vi "CAN Write.vi"(8 "error in (no error)":errorcluster, 10 "MessageBuffer":T1={"ID"=261, "MSGTYPE"=0, "LEN"=8, "DATA[0]"=37, "DATA[1]"=80, "DATA[2]"=37, "DATA[3]"=80, "DATA[4]"=37, "DATA[5]"=80, "DATA[6]"=37, "DATA[7]"=80} {"ID" format="%x"; "MSGTYPE" format="%x"; "LEN" format="%x"; "DATA[0]" format="%x"; "DATA[1]" format="%x"; "DATA[2]" format="%x"; "DATA[3]" format="%x"; "DATA[4]" format="%x"; "DATA[5]" format="%x"; "DATA[6]" format="%x"; "DATA[7]" format="%x"}, 11 "Channel":u16) -> (0 "error out":errorcluster, 2 "MessageBuffer out":T1={"ID"=261, "MSGTYPE"=0, "LEN"=8, "DATA[0]"=37, "DATA[1]"=80, "DATA[2]"=37, "DATA[3]"=80, "DATA[4]"=37, "DATA[5]"=80, "DATA[6]"=37, "DATA[7]"=80} {"ID" format="%x"; "MSGTYPE" format="%x"; "LEN" format="%x"; "DATA[0]" format="%x"; "DATA[1]" format="%x"; "DATA[2]" format="%x"; "DATA[3]" format="%x"; "DATA[4]" format="%x"; "DATA[5]" format="%x"; "DATA[6]" format="%x"; "DATA[7]" format="%x"}, 3 "function return":u32)   [LabVIEW 2020, in "PCANBasic_eX.lvlib"]
doc: "TPCANStatus __stdcall CAN_Write(\n TPCANHandle Channel, \n TPCANMsg* MessageBuffer);"
uses:
  PCANBasic_eX.lvlib
  eX/CTLs/CAN MSG_eX.ctl
  PCANBasic.dll
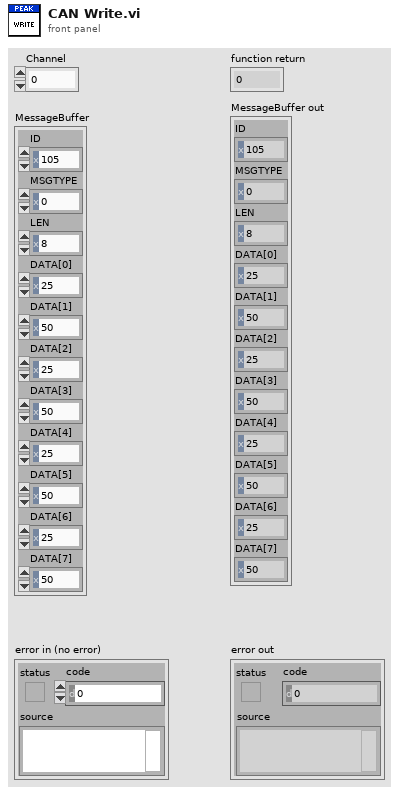
[diagram p1: front panel]
types:
  T1 = typedef "PCANBasic_eX.lvlib/CAN MSG_eX.ctl" = cluster{"ID":u32, "MSGTYPE":u8, "LEN":u8, "DATA[0]":u8, "DATA[1]":u8, "DATA[2]":u8, "DATA[3]":u8, "DATA[4]":u8, "DATA[5]":u8, "DATA[6]":u8, "DATA[7]":u8}
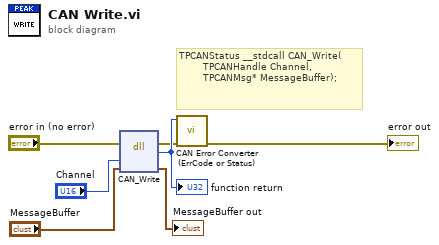
[diagram p0: block diagram]
diagram:
  # "TPCANStatus __stdcall CAN_Write(\n        TPCANHandle Channel, \n        TPCANMsg* MessageBuffer);"
  n1 = dll-call lib="PCANBasic.*" fn="CAN_Write"(error in="error in (no error)", "Channel"="Channel", "MessageBuffer out"="MessageBuffer") -> (error out=w4:errorcluster, w7:u32, "MessageBuffer out"=→"MessageBuffer out":T1)  [unwired: 3 in, 1 out]
  "function return" <- w7
  n2 = call "CAN Error Converter (ErrCode or Status).vi"("error in (no error)"=w4, "error code"=w7) -> ("error out"=→"error out":errorcluster)  [unwired: 9 in]
